vi "Test Write ITX.vi"() -> ()   [LabVIEW 2019, in "LV-Data.ITX.lvclass"]
uses:
  LV-Data.ITX.lvclass
  LV-Data/Typedefs/Dictionary--cluster.ctl
  LV-Data/Typedefs/File Type--enum.ctl
  LV-Data/LV-Data.lvclass
panel:
  out "Data (Dictionary)":T1[](array[typedef])
  out "Array":T1[](array[typedef])
  out "x = y?":cluster{"key":bool, "value":bool}[](array[cluster])
  out "path out":path
  out "XY Graph":cluster{i32[], i32[]}[](graph)
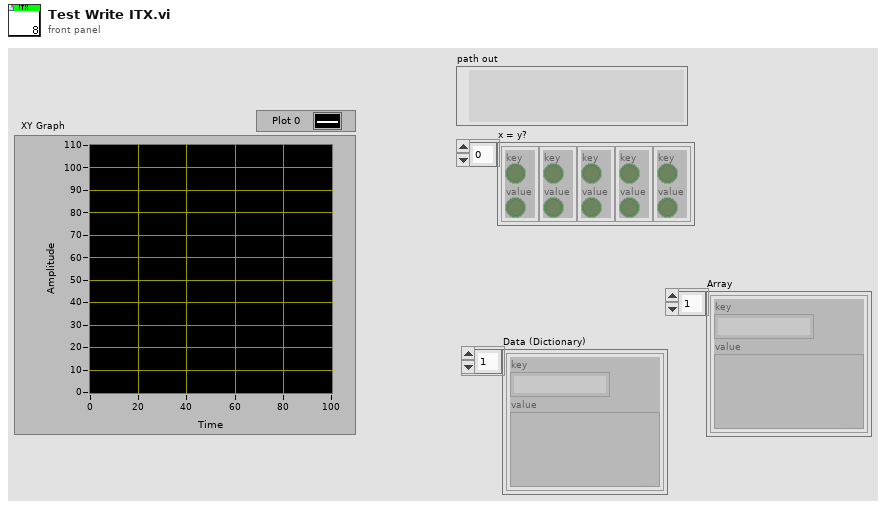
[diagram p1: front panel]
types:
  T1 = typedef "LV-Data.lvclass/Dictionary--cluster.ctl" = cluster{"key":string, "value":variant}
  T2 = typedef "LV-Data.lvclass/File Type--enum.ctl" = enum16{"DAT", "ITX", "TDMS", "VI"}
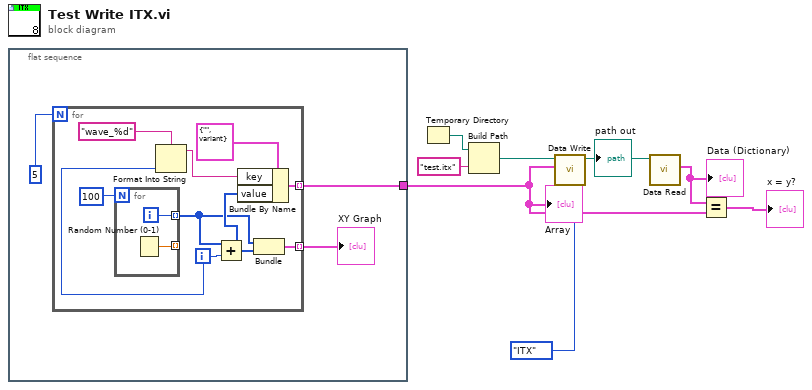
[diagram p0: block diagram]
diagram:
  n1 = flat-sequence {
    tunnel: [w9] -> w2
    frame #0 {
      n2 = for {
        N: 5 -> [_]
        tunnel: [w19] -> w11 mode=indexing
        tunnel: [w14] -> w9 mode=indexing
        i -> [w15]
        n3 = for {
          N: 100 -> [_]
          tunnel: [w22] -> _ mode=indexing
          tunnel: [w21] -> w12 mode=indexing
          i -> [w21]
          n4 = Random Number (0-1)() -> (number: 0 to 1=w22:dbl)
        }
        n5 = Format Into String(format string="wave_%d", w15) -> (resulting string=w16:string)  [unwired: 2 in, 1 out]
        n6 = Add(x=w12, y=w15) -> (x+y=w17:i32[])
        n7 = Bundle By Name(cluster=T1 {"key"="", "value"=variant} ("key-value"), "key"=w16, "value"=w17) -> (w14:T1)
        n8 = Bundle(w12, w17) -> (w19:cluster{i32[], i32[]})  [unwired: 1 in]
      }
      "XY Graph" <- w11
    }
  }
  n9 = Temporary Directory() -> (w7:path)
  n10 = Build Path(base path=w7, name or relative path="test.itx") -> (appended path=w5:path)
  n11 = call "Data Write.vi"("File Type"=File_Type--enum."ITX", "Data (Dictionary)"=w2, "path"=w5) -> ("path out"=w4:path)  [unwired: 7 in, 1 out]
  "path out" <- w4
  n12 = call "Data Read.vi"("path"=w4) -> ("Data (Dictionary)"=w3:T1[])  [unwired: 7 in, 3 out]
  "Data (Dictionary)" <- w3
  n13 = Equal?(x=w3, y=w2) -> (x = y?=→"x = y?":cluster{"key":bool, "value":bool}[])
  "Array" <- w2
